vi "Command (write) - MD.vi"(7 "timeout ms (100)":i32=100, 8 "error in (no error)":errorcluster, 10 "IP":string, 11 "connection ID in":refnum<k16>) -> (0 "error out":errorcluster, 3 "connection ID out":refnum<k16>)   [LabVIEW 2016, in "SMD-7615.lvlib" / "eSCL.lvlib"]
doc: "MD - Motor Disable\nDisables motor outputs (reduces motor current to zero). Disabling the motor also activates the Brake Output function (see BO command). Motor current is not reduced to zero until the Brake Engage (BE command) time has expired."
uses:
  eSCL.lvlib
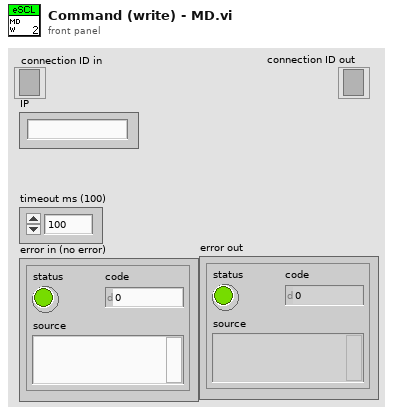
[diagram p1: front panel]
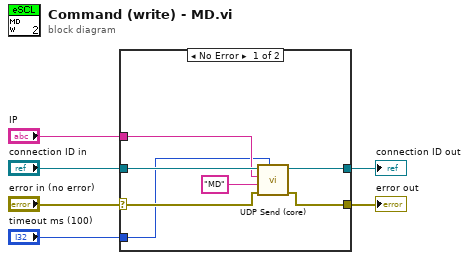
[diagram p0: block diagram]
diagram:
  n1 = case shown="No Error" "error in (no error)" {
    selector: "error in (no error)" -> [w13 w14]
    tunnel: "connection ID in" -> [w12 w15]
    tunnel: [w9 w15] -> w4
    tunnel: [w8 w14] -> w3
    tunnel: "IP" -> [w11 _]
    tunnel: "timeout ms (100)" -> [w10 _]
    frame No Error {
      n2 = call "UDP Send (core).vi"("timeout ms (100)"=w10, "error in (no error)"=w13, "Data"="MD", "IP"=w11, "connection ID in"=w12) -> ("error out"=w8:errorcluster, "connection ID out"=w9:refnum<k16>)  [unwired: 5 in]
    }
    frame Error {
    }
  }
  "connection ID out" <- w4
  "error out" <- w3
